vi "Export - Rx Packet.vi"(8 "error in (no error)":errorcluster, 11 "Device Item Ref in":T4 format="%.0x") -> (0 "error out":errorcluster, 3 "Rx Packet":T1 {"Endianness" items=["big-endian"=0, "little-endian"=2]})   [LabVIEW 2016, in "UDP-Custom-Device System Explorer.lvlib"]
uses:
  UDP-Custom-Device System Explorer.lvlib
  <vilib>/NI Veristand/Custom Device API/Custom Device Item Ref.ctl
  Types/XML - New/ImpExp - Rx Packet Data.ctl
  <vilib>/NI Veristand/Custom Device API/Custom Device Item Info.ctl
  Shared/Types/Shared - Channel Data Type.ctl
  Property Accessors/Shared Packet Accessors.lvlib
  <vilib>/NI VeriStand/Custom Device API/Custom Device API.lvlib
  Property Accessors/Rx Packet Accessors.lvlib
  Shared/UDP-Custom-Device Shared.lvlib
  Property Accessors/Rx Channel Accessors.lvlib
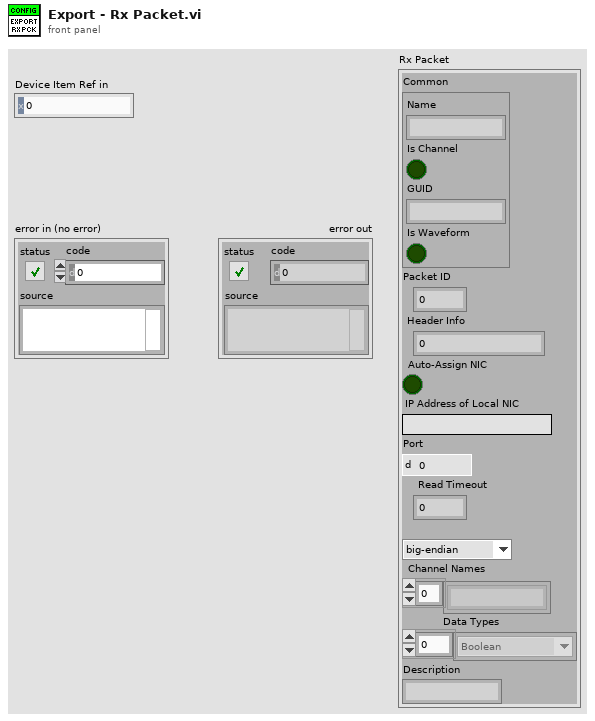
[diagram p1: front panel]
types:
  T1 = typedef "UDP-Custom-Device System Explorer.lvlib/ImpExp - Rx Packet Data.ctl" = cluster{"Common":T2, "Packet ID":i32, "Header Info":u32, "Auto-Assign NIC":bool, "IP Address of Local NIC":string, "Port":u16, "Read Timeout":i32, "Endianness":u16, "Channel Names":string[], "Data Types":T3[], "Description":string}
  T2 = typedef "Custom Device API.lvlib/Custom Device Item Info.ctl" = cluster{"Name":string, "Is Channel":bool, "GUID":string, "Is Waveform":bool}
  T3 = typedef "UDP-Custom-Device Shared.lvlib/Shared - Channel Data Type.ctl" = enum16{"Boolean", "Single", "Double", "I8", "I16", "I32", "I64", "U8", "U16", "U32", "U64"}
  T4 = typedef "Custom Device API.lvlib/Custom Device Item Ref.ctl" = u64
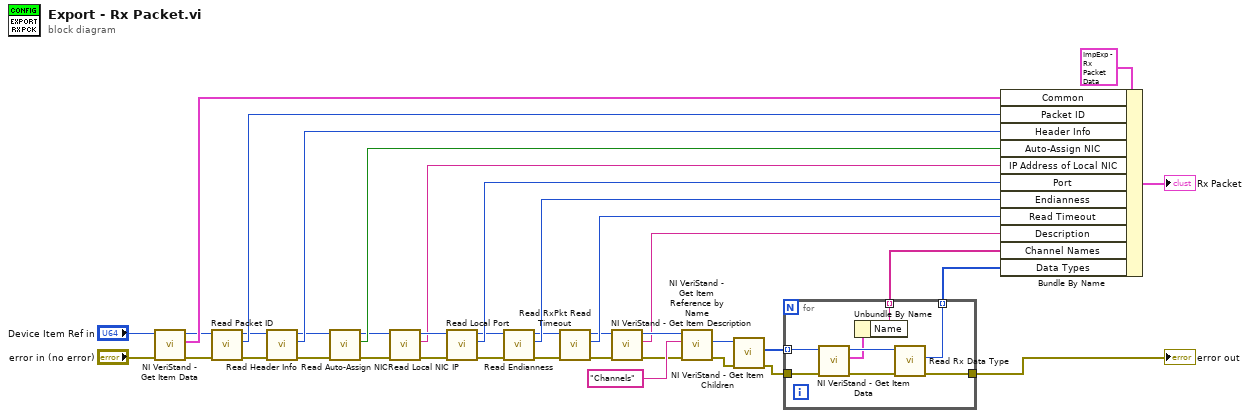
[diagram p0: block diagram]
diagram:
  n1 = call <vilib>:"NI VeriStand - Get Item Data.vi"("error in (no error)"="error in (no error)", "Item Ref in"="Device Item Ref in") -> ("error out"=w20:errorcluster, "Item Info"=w36:T2, "Item Ref out"=w35:T4)  [unwired: 6 in, 1 out]
  n2 = call "Read Packet ID.vi"("error in (no error)"=w20, "Node Ptr"=w35) -> ("error out"=w32:errorcluster, "Packet ID"=w34:i32, "Node Ptr out"=w33:T4)  [unwired: 7 in]
  n3 = call "Read Header Info.vi"("error in (no error)"=w32, "Node Ptr"=w33) -> ("error out"=w29:errorcluster, "Header Info"=w31:u32, "Node Ptr out"=w30:T4)  [unwired: 7 in]
  n4 = call "Read Auto-Assign NIC.vi"("error in (no error)"=w29, "Node Ptr"=w30) -> ("error out"=w24:errorcluster, "Auto-Assign NIC"=w28:bool, "Node Ptr out"=w27:T4)  [unwired: 7 in]
  n5 = call "Read Local NIC IP.vi"("error in (no error)"=w24, "Node Ptr"=w27) -> ("error out"=w25:errorcluster, "IP Address of Local NIC"=w23:string, "Node Ptr out"=w26:T4)  [unwired: 7 in]
  n6 = call "Read Local Port.vi"("error in (no error)"=w25, "Node Ptr"=w26) -> ("error out"=w18:errorcluster, "Port"=w22:u16, "Node Ptr out"=w17:T4)  [unwired: 7 in]
  n7 = call "Read Endianness.vi"("error in (no error)"=w18, "Node Ptr"=w17) -> ("error out"=w15:errorcluster, "Endianness"=w21:u16, "Node Ptr out"=w14:T4)  [unwired: 7 in]
  n8 = call "Read RxPkt Read Timeout.vi"("error in (no error)"=w15, "Node Ptr"=w14) -> ("error out"=w5:errorcluster, "Read Timeout"=w16:i32, "Node Ptr out"=w3:T4)  [unwired: 7 in]
  n9 = call <vilib>:"NI VeriStand - Get Item Description.vi"("error in (no error)"=w5, "Item Ref in"=w3) -> ("error out"=w4:errorcluster, "Description"=w1:string, "Item Ref out"=w2:T4)  [unwired: 6 in, 1 out]
  n10 = call <vilib>:"NI VeriStand - Get Item Reference by Name.vi"("error in (no error)"=w4, "Item Name"="Channels" ("Section Name"), "Parent Ref in"=w2) -> ("error out"=w11:errorcluster, "Item Ref"=w12:T4)  [unwired: 5 in, 2 out]
  n11 = call <vilib>:"NI VeriStand - Get Item Children.vi"("error in (no error)"=w11, "Item Ref in"=w12) -> ("error out"=w9:errorcluster, "Child Refs"=w10:T4[])  [unwired: 6 in, 2 out]
  n12 = for {
    tunnel: w10 -> [w47] mode=indexing
    tunnel: w9 -> [w45]
    tunnel: [w43] -> w8
    tunnel: [w41] -> w7 mode=indexing
    tunnel: [w40] -> w6 mode=indexing
    n13 = call <vilib>:"NI VeriStand - Get Item Data.vi"("error in (no error)"=w45, "Item Ref in"=w47) -> ("error out"=w44:errorcluster, "Item Info"=w42:T2, "Item Ref out"=w46:T4)  [unwired: 6 in, 1 out]
    n14 = Unbundle By Name(w42) -> ("Name"=w41:string)
    n15 = call "Read Rx Data Type.vi"("error in (no error)"=w44, "Node Ptr"=w46) -> ("error out"=w43:errorcluster, "Data Type"=w40:T3)  [unwired: 7 in, 1 out]
  }
  "error out" <- w8
  n16 = Bundle By Name(cluster=T1 {"Common"={"Name"="", "Is Channel"=FALSE, "GUID"="", "Is Waveform"=FALSE}, "Packet ID"=0, "Header Info"=0, "Auto-Assign NIC"=FALSE, "IP Address of Local NIC"="", "Port"=0, "Read Timeout"=0, "Endianness"=0, "Channel Names"=[], "Data Types"=[], "Description"=""} ("Rx Packet"), "Common"=w36, "Packet ID"=w34, "Header Info"=w31, "Auto-Assign NIC"=w28, "IP Address of Local NIC"=w23, "Port"=w22, "Endianness"=w21, "Read Timeout"=w16, "Description"=w1, "Channel Names"=w7, "Data Types"=w6) -> (→"Rx Packet":T1)
